vi "Test Update Table.vi"(4 "error in (no error)":errorcluster, 6 "New Test Record":T2, 7 "Connection Refnum":T1) -> (0 "error out":errorcluster, 3 "Connection Refnum":T1)   [LabVIEW 2011]
uses:
  Test Record.ctl
  SI.LIB/ODBC/SQL Controls/Connection Refnum.ctl
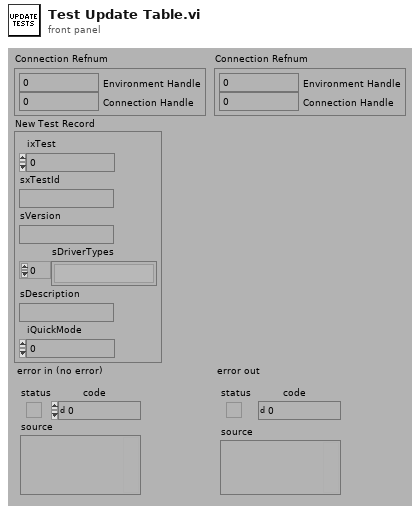
[diagram p1: front panel]
types:
  T1 = typedef "Connection Refnum.ctl" = cluster{"Environment Handle":i32, "Connection Handle":i32}
  T2 = typedef "Test Record.ctl" = cluster{"ixTest":i32, "sxTestId":string, "sVersion":string, "sDriverTypes":string[], "sDescription":string, "iQuickMode":i32}
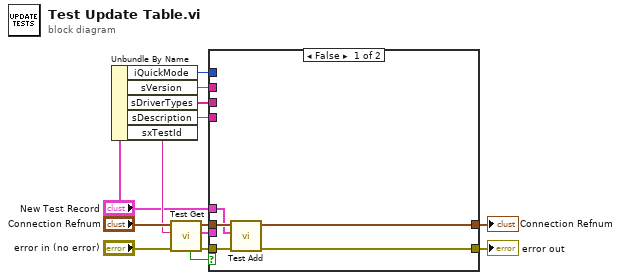
[diagram p0: block diagram]
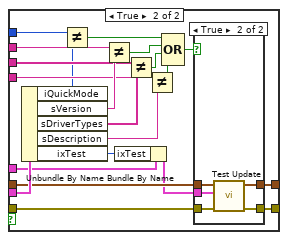
[diagram p2: hidden frame]
diagram:
  n1 = Unbundle By Name("New Test Record") -> ("iQuickMode"=w6:i32, "sVersion"=w12:string, "sDriverTypes"=w11:string[], "sDescription"=w10:string, "sxTestId"=w2:string)
  n2 = call "Test Get.vi"("error in (no error)"="error in (no error)", "Test_ID"=w2, "Connection Refnum"="Connection Refnum") -> ("error out"=w8:errorcluster, "Test Record"=w13:T2, "Connection Refnum"=w9:T1, "Data Present"=w7:bool)  [unwired: 5 out]
  n3 = case shown="False" w7 {
    tunnel: w13 -> [_ w40]
    tunnel: w12 -> [_ w39]
    tunnel: w11 -> [_ w37]
    tunnel: w10 -> [_ w35]
    tunnel: w9 -> [w19 w30]
    tunnel: "New Test Record" -> [w15 w29]
    tunnel: w8 -> [w18 w26]
    tunnel: [w16 w25] -> w3
    tunnel: [w17 w24] -> w5
    tunnel: w6 -> [_ w21]
    frame False {
      n4 = call "Test Add.vi"("error in (no error)"=w18, "Test Record"=w15, "Connection Refnum"=w19) -> ("error out"=w17:errorcluster, "Connection Refnum"=w16:T1)  [unwired: 7 out]
    }
    frame True {
      n5 = Unbundle By Name(w40) -> ("iQuickMode"=w22:i32, "sVersion"=w38:string, "sDriverTypes"=w36:string[], "sDescription"=w34:string, "ixTest"=w28:i32)
      n6 = Not Equal?(x=w21, y=w22) -> (x != y?=w20:bool)
      n7 = Not Equal?(x=w39, y=w38) -> (x != y?=w33:bool)
      n8 = Bundle By Name(cluster=w29, "ixTest"=w28) -> (w27:T2)
      n9 = Not Equal?(x=w37, y=w36) -> (x != y?=w32:bool)
      n10 = Not Equal?(x=w35, y=w34) -> (x != y?=w31:bool)
      n11 = Compound Arithmetic op=OR(w20, w33, w32, w31) -> (w23:bool)
      n12 = case shown="True" w23 {
        tunnel: w30 -> [w42 w47]
        tunnel: w27 -> [_ w46]
        tunnel: w26 -> [w41 w45]
        tunnel: [w42 w44] -> w25
        tunnel: [w41 w43] -> w24
        frame False {
        }
        frame True {
          n13 = call "Test Update.vi"("error in (no error)"=w45, "Test Record"=w46, "Connection Refnum"=w47) -> ("error out"=w43:errorcluster, "Connection Refnum"=w44:T1)  [unwired: 7 out]
        }
      }
    }
  }
  "error out" <- w5
  "Connection Refnum" <- w3
